vi "calcStiffnesses.vi"(8 "error in (no error)":errorcluster, 11 "StiffnessCalculator in":refnum<class "StiffnessCalculator.lvclass">) -> (0 "error out":errorcluster, 3 "StiffnessCalculator out":refnum<class "StiffnessCalculator.lvclass">)   [LabVIEW 2015, in "StiffnessCalculator.lvclass"]
uses:
  StiffnessCalculator.lvclass
  StiffnessCalculator.lvclass/StiffnessCalculator.ctl
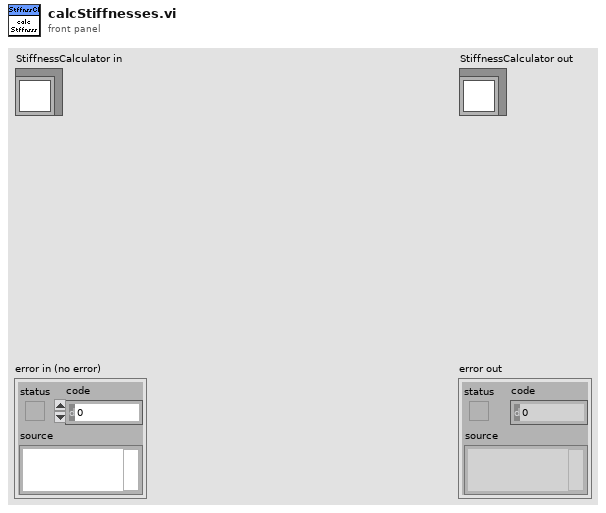
[diagram p1: front panel]
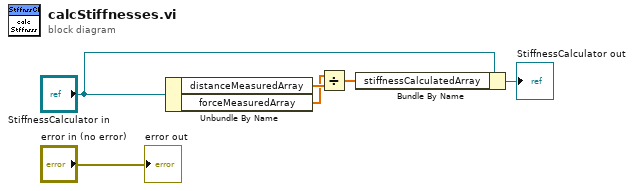
[diagram p0: block diagram]
diagram:
  n1 = Unbundle By Name("StiffnessCalculator in") -> ("distanceMeasuredArray"=w3:dbl[unit][], "forceMeasuredArray"=w2:dbl[unit][])
  n2 = Divide(x=w2, y=w3) -> (x/y=w1:dbl[unit][])
  n3 = Bundle By Name(cluster="StiffnessCalculator in", "stiffnessCalculatedArray"=w1) -> (→"StiffnessCalculator out":refnum<class "StiffnessCalculator.lvclass">)
  "error out" <- "error in (no error)"
